vi "Initialize.vi"() -> ()   [LabVIEW 2018]
panel:
  out "Save Path Out":path
  in  "Save Path In":path
  out "DLL Path Out":path
  in  "DLL Path In":path
  # "GPU CUDA -"
  # "INITIALIZE"
  # "Path to CUDA DLL"
  # "Path To Save GPU & Core Errors Info"
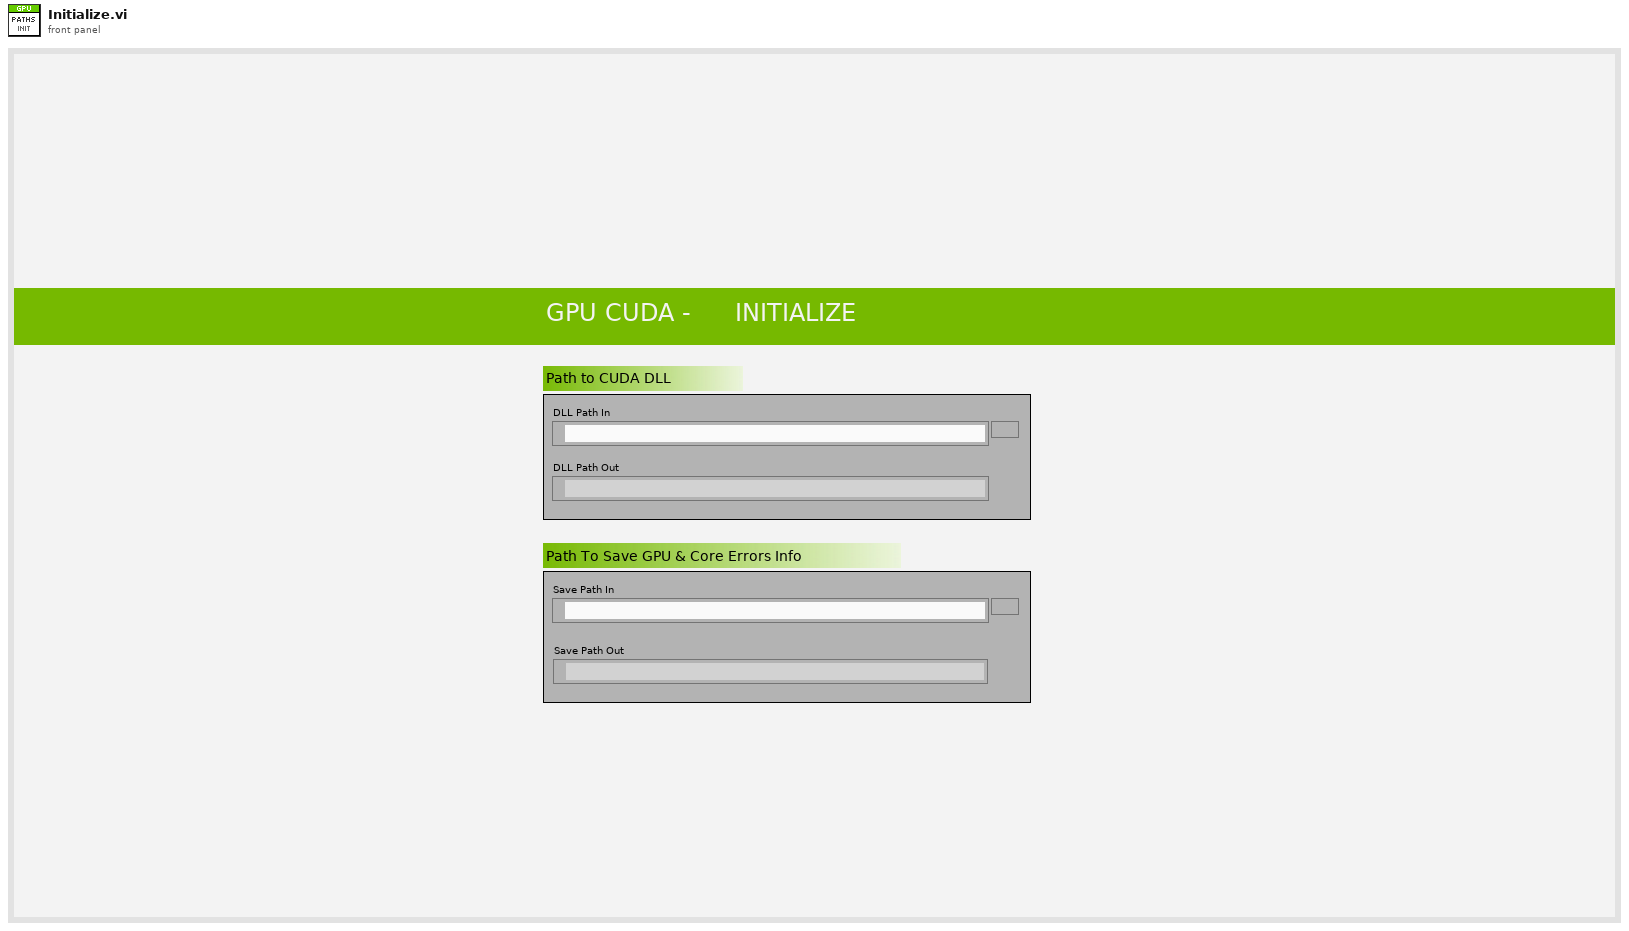
[diagram p1: front panel]
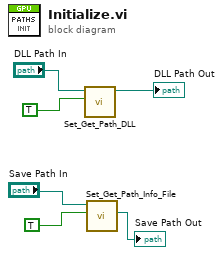
[diagram p0: block diagram]
diagram:
  n1 = call "Set_Get_Path_DLL.vi"("Add Path DLL (False)"=TRUE, "path DLL"="DLL Path In") -> ("path DLL Out"=→"DLL Path Out":path)  [unwired: 9 in]
  n2 = call "Set_Get_Path_Info_File.vi"("Add Info File Path (False)"=TRUE, "Info File Path"="Save Path In") -> ("Info File Path Out"=→"Save Path Out":path)  [unwired: 8 in, 1 out]
